vi "ziGetEventDIOSample.vi"(8 "Error In":errorcluster, 10 "DIOIn":T1, 11 "Handle In":T2 {"Handle" format="0x%08x"; "Conn" format="0x%08x"}) -> (0 "Error Out":errorcluster, 2 "DIO Out":T1, 3 "Handle Out":T2 {"Handle" format="0x%08x"; "Conn" format="0x%08x"})   [LabVIEW 2018, in "Zurich Instruments LabOne.lvlib"]
uses:
  Zurich Instruments LabOne.lvlib
  <instrlib>/Zurich Instruments LabOne/Private/ziLV64.framework
  ziTypeHandle.ctl
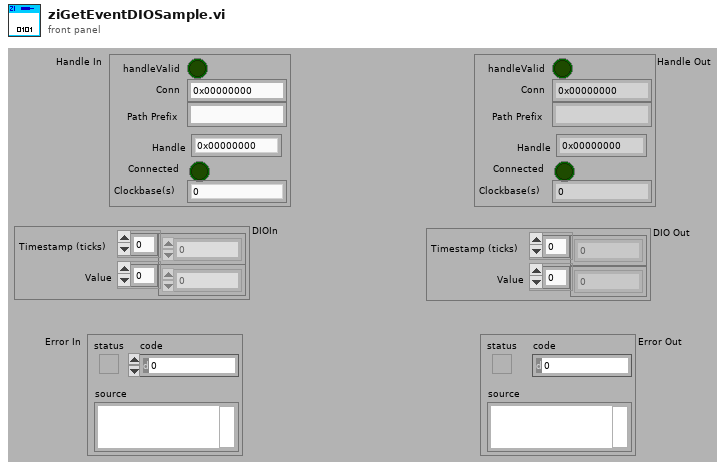
[diagram p1: front panel]
types:
  T1 = cluster{"Timestamp (ticks)":u64[], "Value":u32[]}
  T2 = typedef "Zurich Instruments LabOne.lvlib/ziTypeHandle.ctl" = cluster{"handleValid":bool, "Conn":u64, "Path Prefix":string, "Handle":u64, "Connected":bool, "Clockbase(s)":dbl}
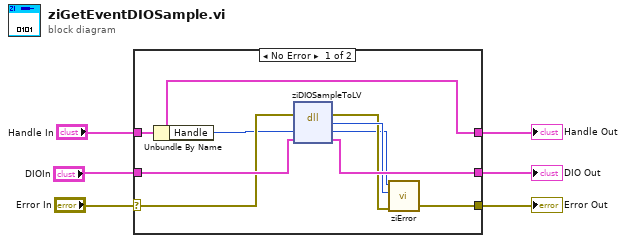
[diagram p0: block diagram]
diagram:
  n1 = case shown="No Error" "Error In" {
    selector: "Error In" -> [w12 w16]
    tunnel: "Handle In" -> [w8 w18]
    tunnel: [w8 w18] -> w5
    tunnel: [w15 w16] -> w4
    tunnel: [w14 w17] -> w3
    tunnel: "DIOIn" -> [w13 w17]
    frame No Error {
      n2 = Unbundle By Name(w8) -> ("Handle"=w11:u64)
      n3 = dll-call lib="Applications/National Instruments/LabVIEW 2019 64-bit/instr.lib/Zurich Instruments LabOne/Private/ziLV*.*" fn="ziDIOSampleToLV"(error in=w12, "ziEventBuffer"=w11, "Sample"=w13) -> (error out=w9:errorcluster, "return type"=w10:u32, "ziEventBuffer"=w7:u64, "Sample"=w14:T1)  [unwired: 2 in, 1 out]
      n4 = call "ziError.vi"("Conn"=w7, "ziErrorCode"=w10, "Error In"=w9) -> ("Error Out"=w15:errorcluster)  [unwired: 2 in, 1 out]
    }
    frame Error {
    }
  }
  "Handle Out" <- w5
  "Error Out" <- w4
  "DIO Out" <- w3
